vi "GetSlitwidth.vi"(8 "error in (no error)":errorcluster, 10 "Slit":T1(ring), 11 "DongWoo in":refnum<class "DongWoo.lvclass">) -> (0 "error out":errorcluster, 3 "DongWoo out":refnum<class "DongWoo.lvclass">)   [LabVIEW 2023, in "DongWoo_Spectrometer.lvlib" / "DongWoo.lvclass"]
uses:
  DongWoo.lvclass
  DongWoo.lvclass/DongWoo.ctl
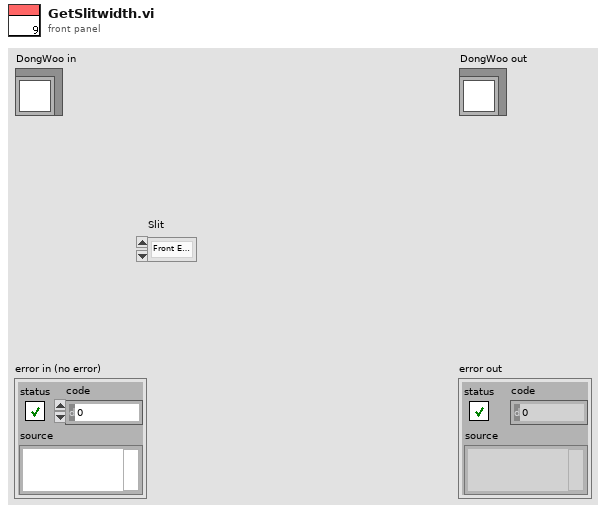
[diagram p1: front panel]
types:
  T1 = enum16{"Front Entrance Slit", "Side Entrance Slit", "Front Exit Slit", "Side Exit Slit"}
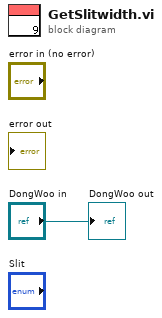
[diagram p0: block diagram]
diagram:
  "DongWoo out" <- "DongWoo in"
